vi "Add Log Handler.vi"(8 "error in (no error)":errorcluster, 10 "Log Handler":refnum<class "Logging.lvclass">, 11 "Process In":refnum<class "Process.lvclass">) -> (0 "error out":errorcluster, 3 "Process Out":refnum<class "Process.lvclass">)   [LabVIEW 2020, in "Process.lvclass"]
uses:
  Process.lvclass
  Logging/Logging.lvclass
  Process.lvclass/Process.ctl
  <vilib>/Utility/error.llb/Clear Errors.vi
  <vilib>/Utility/error.llb/Error Cluster From Error Code.vi
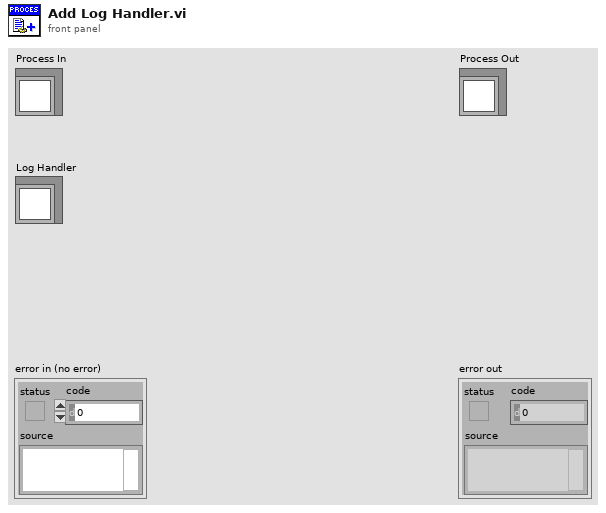
[diagram p1: front panel]
types:
  T1 = typedef "Process.lvclass/Lifecycle State.ctl" = enum16{"Uninitialized", "Initialized", "Started", "Running", "Stopped", "Finished"}
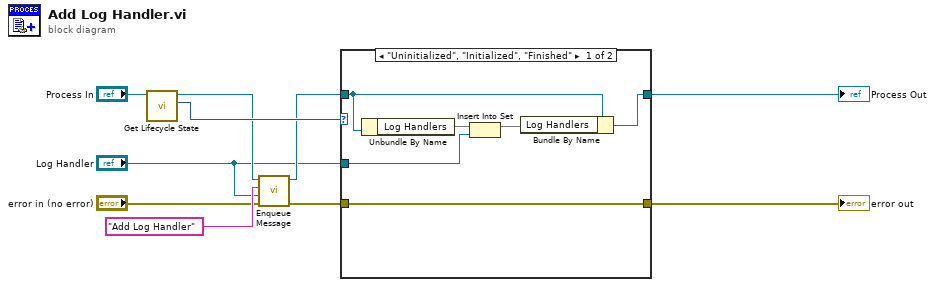
[diagram p0: block diagram]
diagram:
  n1 = call "Get Lifecycle State.vi"("Process In"="Process In") -> ("Lifecycle State"=w9:T1, "Process Out"=w5:refnum<class "Process.lvclass">)  [unwired: 7 in, 2 out]
  n2 = call "Enqueue Message.vi"("error in (no error)"="error in (no error)", "Message Data"="Log Handler", "Message"="Add Log Handler", "Process In"=w5) -> ("error out"=w6:errorcluster, "Process Out"=w4:refnum<class "Process.lvclass">)  [unwired: 6 in]
  n3 = case shown="\"Uninitialized\", \"Initialized\", \"Finished\"" w9 {
    tunnel: "Log Handler" -> [w11 _]
    tunnel: [w13 w18] -> w8
    tunnel: [w12 w17] -> w7
    tunnel: w6 -> [w13 w18]
    tunnel: w4 -> [w14 w17]
    frame "Uninitialized", "Initialized", "Finished" {
      n4 = Unbundle By Name(w14) -> ("Log Handlers"=w15:set{refnum<class "Logging.lvclass">})
      n5 = Insert Into Set(10:w11, 11:w15) -> (3:w16:set{refnum<class "Logging.lvclass">})  [unwired: 1 out]
      n6 = Bundle By Name(cluster=w14, "Log Handlers"=w16) -> (w12:refnum<class "Process.lvclass">)
    }
    frame "Started".."Stopped" {
    }
  }
  "error out" <- w8
  "Process Out" <- w7
